vi "get_segments.vi"(8 "error in (no error)":errorcluster, 9 "range":dbl[unit], 10 "offset":dbl[unit], 11 "GenericTrajectory in":refnum<class "TrajectoryDL091126GenericVoxel.lvclass">) -> (0 "error out":errorcluster, 2 "segments":T1[](array[typedef]), 3 "GenericTrajectory out":refnum<class "TrajectoryDL091126GenericVoxel.lvclass">)   [LabVIEW 2010, in "TrajectoryDL091126GenericVoxel.lvclass"]
uses:
  TrajectoryDL091126GenericVoxel.lvclass
  segment_cluster.ctl
  common/enumerations/x_y_z_enumeration.ctl
  common/enumerations/functional_global_action_enum.ctl
  common/classes/ErrorController/ErrorController/class_data.vi
  common/classes/ErrorController/ErrorController/ErrorController.lvclass
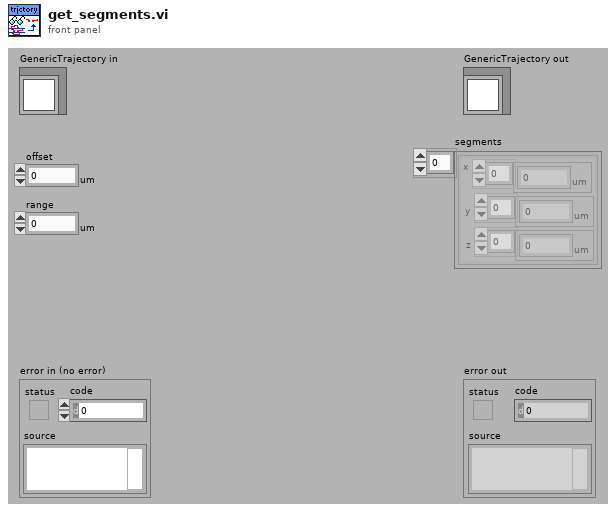
[diagram p1: front panel]
types:
  T1 = typedef "TrajectoryDL091126GenericVoxel.lvclass/segment_cluster.ctl" = cluster{"x":dbl[unit][], "y":dbl[unit][], "z":dbl[unit][]}
  T2 = typedef "x_y_z_enumeration.ctl" = enum16{"x", "y", "z"}
  T3 = typedef "functional_global_action_enum.ctl" = enum16{"get", "set", "reset"}
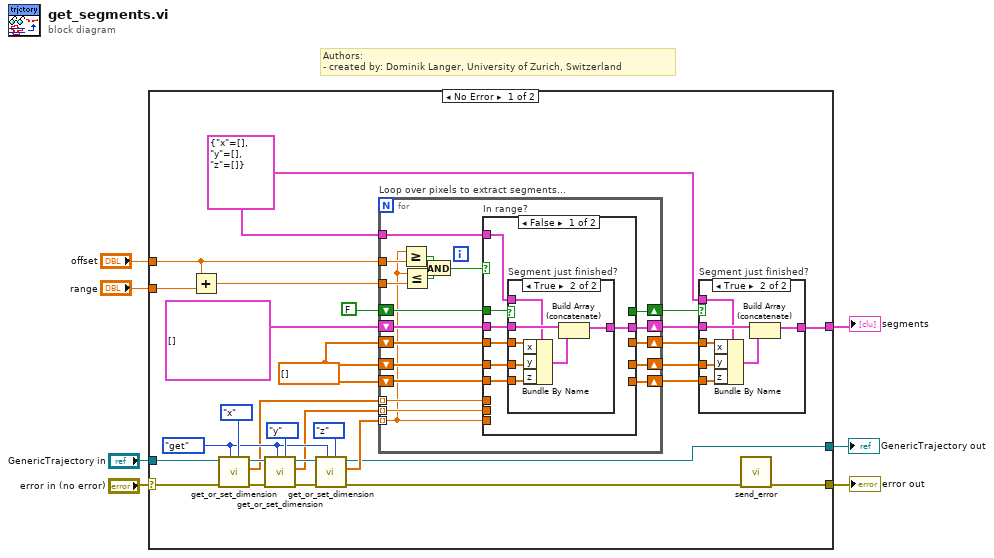
[diagram p0: block diagram]
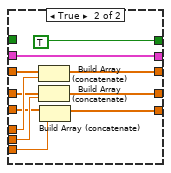
[diagram p4: hidden frame]
diagram:
  # "Authors: \n- created by: Dominik Langer, University of Zurich, Switzerland"
  n1 = case shown="No Error" "error in (no error)" {
    selector: "error in (no error)" -> [w32 w91]
    tunnel: [w9 w91] -> w6
    tunnel: [w8 w90] -> w4
    tunnel: "GenericTrajectory in" -> [w11 w90]
    tunnel: "offset" -> [w22 _]
    tunnel: "range" -> [w24 _]
    tunnel: [w12 _] -> w1
    frame No Error {
      w13 = T1 {"x"=[], "y"=[], "z"=[]} ("segment")
      w21 = dbl[unit][] []
      w30 = functional_global_action_enum."get" ("action")
      n2 = Add(x=w22, y=w24) -> (x+y=w23:dbl[unit])
      n3 = call-dynamic "get_or_set_dimension.vi"("dimension"=x_y_z_enumeration."x", "action"=w30, "error in (no error)"=w32, "GenericTrajectory in"=w11) -> ("error out"=w34:errorcluster, "pixel values out (single dimension)"=w27:dbl[unit][], "GenericTrajectory out"=w33:refnum<class "TrajectoryDL091126GenericVoxel.lvclass">)  [unwired: 5 in]
      n4 = call-dynamic "get_or_set_dimension.vi"("dimension"=x_y_z_enumeration."y", "action"=w30, "error in (no error)"=w34, "GenericTrajectory in"=w33) -> ("error out"=w31:errorcluster, "pixel values out (single dimension)"=w26:dbl[unit][], "GenericTrajectory out"=w28:refnum<class "TrajectoryDL091126GenericVoxel.lvclass">)  [unwired: 5 in]
      n5 = call-dynamic "get_or_set_dimension.vi"("dimension"=x_y_z_enumeration."z", "action"=w30, "error in (no error)"=w31, "GenericTrajectory in"=w28) -> ("error out"=w10:errorcluster, "pixel values out (single dimension)"=w25:dbl[unit][], "GenericTrajectory out"=w8:refnum<class "TrajectoryDL091126GenericVoxel.lvclass">)  [unwired: 5 in]
      n6 = for "Loop over pixels to extract segments..." {
        tunnel: w27 -> [w60] mode=indexing
        tunnel: w26 -> [w57] mode=indexing
        tunnel: w25 -> [w45] mode=indexing
        tunnel: w23 -> [w46]
        tunnel: w22 -> [w63]
        shift-right: [w61] -> w17
        shift-left: w21 -> [w62]
        shift-right: [w59] -> w16
        shift-left: w21 -> [w58]
        shift-right: [w56] -> w15
        shift-left: w21 -> [w55]
        shift-right: [w54] -> w18
        shift-left: FALSE -> [w52]
        shift-right: [w50] -> w14
        shift-left: T1[] [] ("segments") -> [w53]
        tunnel: w13 -> [w51]
        n7 = Greater Or Equal?(x=w45, y=w63) -> (x >= y?=w47:bool)
        n8 = Less Or Equal?(x=w45, y=w46) -> (x <= y?=w48:bool)
        n9 = And(x=w47, y=w48) -> (x .and. y?=w49:bool)
        n10 = case "In range?" shown="False" w49 {
          tunnel: w62 -> [w68 w89]
          tunnel: [_ w88] -> w61
          tunnel: w60 -> [_ w87]
          tunnel: [_ w86] -> w59
          tunnel: w58 -> [w67 w85]
          tunnel: w57 -> [_ w84]
          tunnel: w45 -> [_ w83]
          tunnel: [_ w82] -> w56
          tunnel: w55 -> [w66 w81]
          tunnel: [_ TRUE] -> w54
          tunnel: w53 -> [w70 w79]
          tunnel: w52 -> [w64 _]
          tunnel: w51 -> [w69 _]
          tunnel: [w65 w79] -> w50
          frame False {
            n11 = case "Segment just finished?" shown="True" w64 {
              tunnel: w70 -> [w71 w78]
              tunnel: w69 -> [_ w77]
              tunnel: w68 -> [_ w76]
              tunnel: w67 -> [_ w75]
              tunnel: w66 -> [_ w74]
              tunnel: [w71 w72] -> w65
              frame False {
              }
              frame True {
                n12 = Bundle By Name(cluster=w77, "x"=w76, "y"=w75, "z"=w74) -> (w73:T1)
                n13 = Build Array (concatenate)(w78, w73) -> (w72:T1[])
              }
            }
          }
          frame True {
            n14 = Build Array (concatenate)(w89, w87) -> (w88:dbl[unit][])
            n15 = Build Array (concatenate)(w85, w84) -> (w86:dbl[unit][])
            n16 = Build Array (concatenate)(w81, w83) -> (w82:dbl[unit][])
          }
        }
      }
      n17 = case "Segment just finished?" shown="True" w18 {
        tunnel: w14 -> [w37 w44]
        tunnel: w13 -> [_ w43]
        tunnel: w17 -> [_ w42]
        tunnel: w16 -> [_ w41]
        tunnel: w15 -> [_ w40]
        tunnel: [w37 w38] -> w12
        frame False {
        }
        frame True {
          n18 = Bundle By Name(cluster=w43, "x"=w42, "y"=w41, "z"=w40) -> (w39:T1)
          n19 = Build Array (concatenate)(w44, w39) -> (w38:T1[])
        }
      }
      n20 = call "send_error.vi"("error in (no error)"=w10) -> ("error out"=w9:errorcluster)  [unwired: 10 in]
    }
    frame Error {
    }
  }
  "error out" <- w6
  "GenericTrajectory out" <- w4
  "segments" <- w1
